vi "Randomize Array (LabVIEW 2021).vi"() -> ()   [LabVIEW 2021]
panel:
  out "Randomized Array":dbl[](array[numeric])
  in  "Array":dbl[](array[numeric])
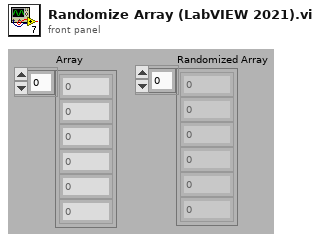
[diagram p1: front panel]
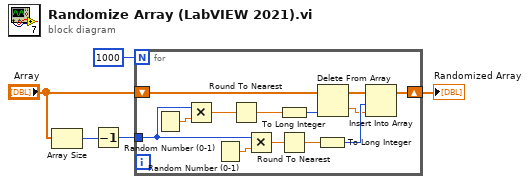
[diagram p0: block diagram]
diagram:
  n1 = Array Size(array="Array") -> (size(s)=w3:i32)
  n2 = Decrement(x=w3) -> (x-1=w2:i32)
  n3 = for {
    N: 1000 -> [_]
    shift-right: [w7] -> w1
    shift-left: "Array" -> [w10]
    tunnel: w2 -> [w18]
    n4 = Random Number (0-1)() -> (number: 0 to 1=w17:dbl)
    n5 = Multiply(x=w18, y=w17) -> (x*y=w16:dbl)
    n6 = Random Number (0-1)() -> (number: 0 to 1=w6:dbl)
    n7 = Round To Nearest(number=w16) -> (nearest integer value=w14:dbl)
    n8 = Multiply(x=w18, y=w6) -> (x*y=w15:dbl)
    n9 = To Long Integer(number=w14) -> (32bit integer=w11:i32)
    n10 = Round To Nearest(number=w15) -> (nearest integer value=w13:dbl)
    n11 = To Long Integer(number=w13) -> (32bit integer=w12:i32)
    n12 = Delete From Array(array=w10, index=w11) -> (deleted portion=w8:dbl, array with subset deleted=w9:dbl[])  [unwired: 1 in]
    n13 = Insert Into Array(array=w9, index=w12, new element=w8) -> (w7:dbl[])
  }
  "Randomized Array" <- w1
